vi "Dequeue Command.vi"(7 "Wait? (T)":bool=TRUE, 8 "error in (no error)":errorcluster, 11 "VISA Client in":refnum<class "Serial Client.lvclass">) -> (0 "error out":errorcluster, 1 "Timed Out":bool, 2 "Command":T1, 3 "VISA Client out":refnum<class "Serial Client.lvclass">)   [LabVIEW 2020, in "Stream-Serial.lvlib" / "Serial Client.lvclass"]
uses:
  Serial Client.lvclass
  Client Command.ctl
  Serial Client.lvclass/Serial Client.ctl
  Stream-Serial.lvlib
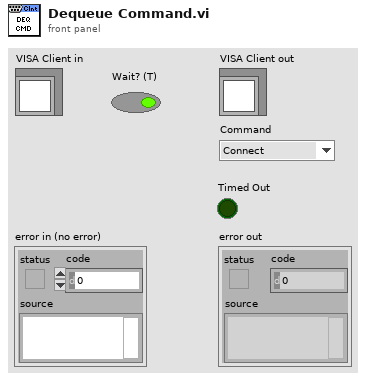
[diagram p1: front panel]
types:
  T1 = typedef "Stream-Serial.lvlib/Client Command.ctl" = enum16{"Connect", "Close", "Shutdown", "Reconnect"}
  T2 = typedef "Stream-Serial.lvlib/Command Queue.ctl" = refnum<queue>
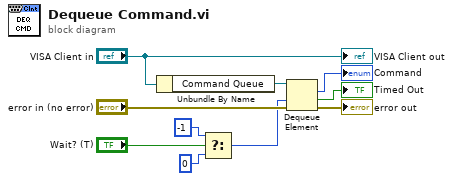
[diagram p0: block diagram]
diagram:
  n1 = Unbundle By Name("VISA Client in") -> ("Command Queue"=w6:T2)
  n2 = Select(t=-1, s="Wait? (T)", f=0) -> (s? t:f=w4:i32)
  n3 = Dequeue Element(queue=w6, timeout in ms (-1)=w4, error in (no error)="error in (no error)") -> (element=→"Command":T1, timed out?=→"Timed Out":bool, error out=→"error out":errorcluster)  [unwired: 1 out]
  "VISA Client out" <- "VISA Client in"
